vi "Save_v5.vi"(8 "error in":errorcluster, 9 "Save Cluster":T1={"Version"="", "Devices"=[], "Select Layout"=0, "Layout:Strings And Values []"=[], "User defined functions"="-- -------------------------------------------------------------------------------------------\n-- The following functions are part of the \"standard load\" of functions and should not be messed with\n-- They are here for reference only.\n-- Please add any user functions above this comment\n-- -------------------------------------------------------------------------------------------\n\n-- Creates a linear ramp from A to B\nfunction LineRamp(f, Initial, Final)\n    return (1-f)*Initial + f*Final;\nend\n\n-- Creates an exponential ramp from A to B\nfunction ExpRamp(t, a, b, tau)\n   return (b - a*exp(tMax / tau) + (a-b)*exp(t/tau))/ ( 1 - exp(tMax / tau) );\nend\n\n-- Creates a sinewave\nfunction SinRamp(t,Offset,A,Freq, Phase)\n    return Offset + A * sin(2*pi*Freq*t + Phase)\nend\n\n-- Creates a blackman pulse\nfunction Blackman(f, Offset, A)\n    return Offset +  A*sqrt(0.5*cos(3.1415*(2*f-1))+0.08*cos(2*pi*(2*f-1))+0.42);\nend\n\n-- Creates a half-gauss ramp\nfunction HalfGaussRamp(t, a, b, Width)\n    local y;\n    y = exp(-(tMax^2)/Width^2);\n    y = (a -  b*y)/(1-y)  +  ((b-a)/(1-y))*exp(-((t-tMax)^2)/Width^2);\n    return y;\nend\n\n-- Creates an \"O'Hara\" ramp from A to B, for dipole evaporation\nfunction EvapRamp(t, a, b, tau)\n   local y;\n  y = log(a/b) / log(1+tMax/tau);\n  y = a * (1+t/tau)^(-y);\n  return y;\nend\n", "VariableManager"=refnum} {"Select Layout" items=["Default"]}, 11 "Path (open dialog)":path) -> (0 "error out":errorcluster, 1 "cancelled":bool, 2 "Procedure Name":string, 3 "Chosen Path":path)   [LabVIEW 2013]
doc: "Save entire SetList configuration to disk. This includes Device configuration, software image, user procedures, variables, layouts.\n\nIf no \"path\" to file is given, the user is presented with a dialog box. The chosen full path is returned, as well as the file name as \"Procedure Name.\""
uses:
  TypeDefs/SaveCluster.ctl
  VariableManagerCodes/VariableManager/VariableManager.lvclass
  DeviceVIs/Device/Device.lvclass
  <vilib>/Utility/miscctls.llb/LVStringsAndValuesArrayTypeDef_I32.ctl
panel:
  # "note: if user cancels, will also throw an\nerror (code 43)"
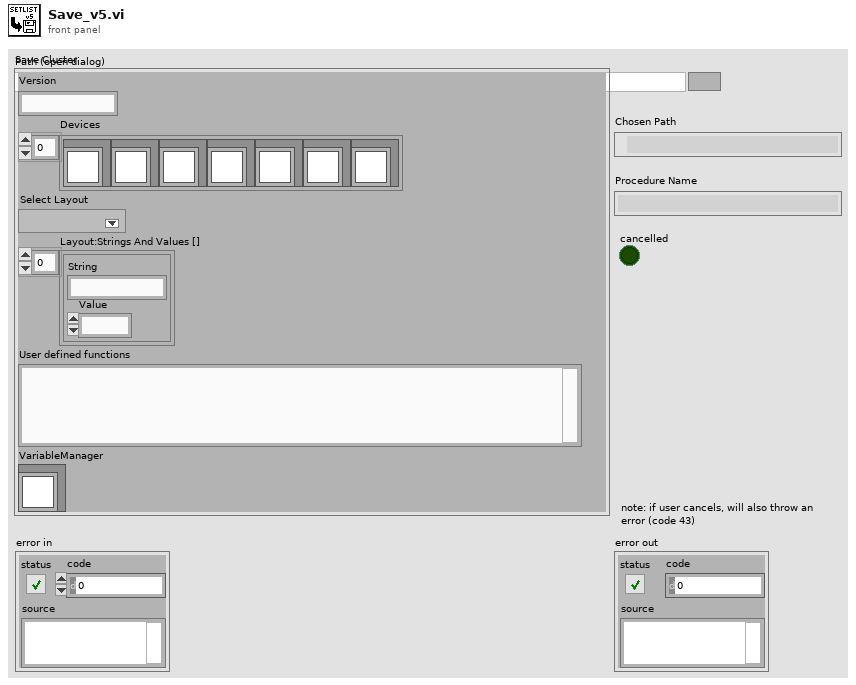
[diagram p1: front panel]
types:
  T1 = typedef "SaveCluster.ctl" = cluster{"Version":string, "Devices":refnum<class "Device.lvclass">[], "Select Layout":i32, "Layout:Strings And Values []":T2, "User defined functions":string, "VariableManager":refnum<class "VariableManager.lvclass">}
  T2 = typedef "LVStringsAndValuesArrayTypeDef_I32.ctl" = cluster{"String":string, "Value":i32}[]
  T3 = enum16{"open", "replace", "create", "open or create", "replace or create", "replace or create with confirmation"}
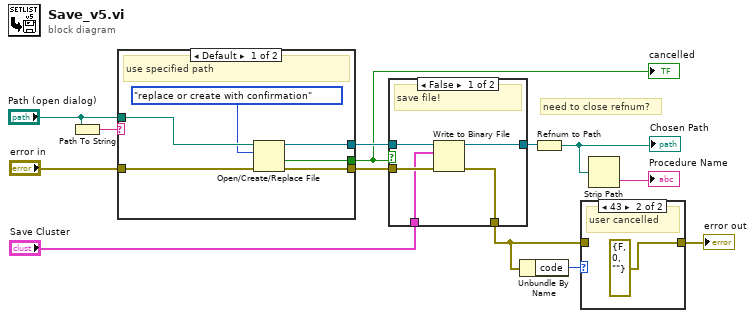
[diagram p0: block diagram]
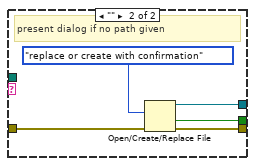
[diagram p4: hidden frame]
diagram:
  # "need to close refnum?"
  n1 = Path To String(path="Path (open dialog)") -> (string=w13:string)
  n2 = case shown="Default" w13 {
    tunnel: "Path (open dialog)" -> [w19 _]
    tunnel: "error in" -> [w17 w23]
    tunnel: [w15 w21] -> w7
    tunnel: [w16 w22] -> w9
    tunnel: [w14 w20] -> w10
    frame Default {
      # "use specified path"
      n3 = Open/Create/Replace File(file path (use dialog)=w19, error in=w17, operation (0:open)=T3."replace or create with confirmation") -> (refnum out=w14:refnum<file>, cancelled=w15:bool, error out=w16:errorcluster)  [unwired: 3 in]
    }
    frame "" {
      # "present dialog if no path given"
      n4 = Open/Create/Replace File(error in=w23, operation (0:open)=T3."replace or create with confirmation") -> (refnum out=w20:refnum<file>, cancelled=w21:bool, error out=w22:errorcluster)  [unwired: 4 in]
    }
  }
  "cancelled" <- w7
  n5 = case shown="False" w7 {
    tunnel: [w25 w31] -> w6
    tunnel: [w29 w30] -> w2
    tunnel: w10 -> [w28 w31]
    tunnel: w9 -> [w27 w30]
    tunnel: "Save Cluster" -> [w26 _]
    frame False {
      # "save file!"
      n6 = Write to Binary File(file (use dialog)=w28, data=w26, error in=w27) -> (refnum out=w25:refnum<file>, error out=w29:errorcluster)  [unwired: 3 in, 1 out]
    }
    frame True {
      # "user cancelled"
    }
  }
  n7 = Unbundle By Name(w2) -> ("code"=w3:i32)
  n8 = Refnum to Path(1:w6) -> (0:w5:path)
  "Chosen Path" <- w5
  n9 = case shown="43" w3 {
    tunnel: w2 -> [w32 _]
    tunnel: [w32 errorcluster {"status"=FALSE, "code"=0, "source"=""} ("error out")] -> w1
    frame Default {
      # "pass other"
    }
    frame 43 {
      # "user cancelled"
    }
  }
  "error out" <- w1
  n10 = Strip Path(path=w5) -> (name=→"Procedure Name":string)  [unwired: 1 out]
